vi "RIOchannelStorage.vi"(8 "Error in":errorcluster, 10 "Channel Settings":T1[][](array[typedef]), 11 "Tree DVR in":refnum<data-value>) -> (0 "Error out":errorcluster)   [LabVIEW 2014]
uses:
  Controls/RIOSettingsChannelSettings.ctl
  <vilib>/MDSplus/Classes/Tree_Class/Tree.lvclass
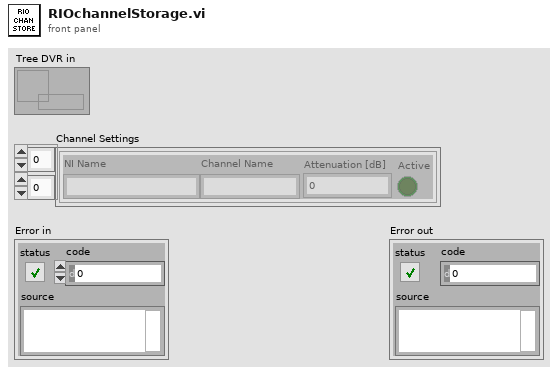
[diagram p1: front panel]
types:
  T1 = typedef "RIOSettingsChannelSettings.ctl" = cluster{"Channel Name":string, "Active":bool, "NI Name":string, "Attenuation [dB]":i32}
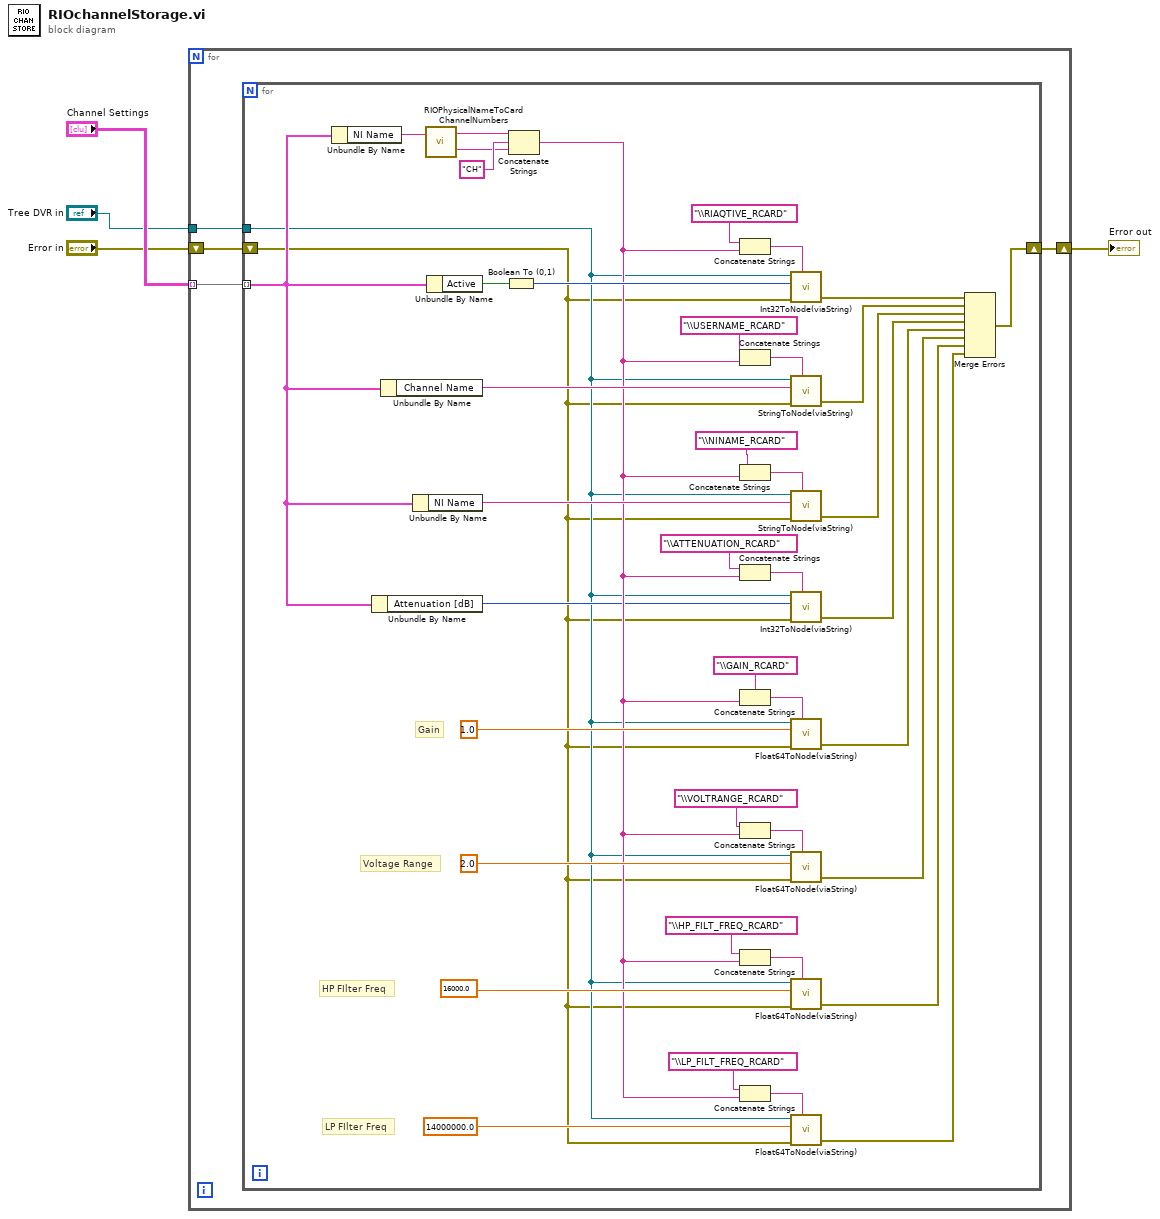
[diagram p0: block diagram]
diagram:
  n1 = for {
    tunnel: "Channel Settings" -> [w8] mode=indexing
    shift-right: [w7] -> w2
    shift-left: "Error in" -> [w5]
    tunnel: "Tree DVR in" -> [w6]
    n2 = for {
      tunnel: w8 -> [w17] mode=indexing
      tunnel: w6 -> [w15]
      shift-right: [w50] -> w7
      shift-left: w5 -> [w14]
      # "LP FIlter Freq"
      # "Voltage Range"
      # "HP FIlter Freq"
      # "Gain"
      n3 = Unbundle By Name(w17) -> ("NI Name"=w21:string)
      n4 = Unbundle By Name(w17) -> ("Attenuation [dB]"=w16:i32)
      n5 = Unbundle By Name(w17) -> ("Channel Name"=w28:string)
      n6 = Unbundle By Name(w17) -> ("NI Name"=w27:string)
      n7 = call "RIOPhysicalNameToCardChannelNumbers.vi"("Channel Name"=w21) -> ("Channel #"=w22:string, "Card #"=w23:string)  [unwired: 1 in]
      n8 = Unbundle By Name(w17) -> ("Active"=w47:bool)
      n9 = Boolean To (0,1)(Boolean=w47) -> (0, 1=w46:i16)
      n10 = Concatenate Strings(w23, "CH" ("string"), w22) -> (w18:string)
      n11 = Concatenate Strings("\\RIAQTIVE_RCARD" ("string"), w18) -> (w44:string)
      n12 = Concatenate Strings("\\USERNAME_RCARD" ("string"), w18) -> (w31:string)
      n13 = Concatenate Strings("\\NINAME_RCARD" ("string"), w18) -> (w29:string)
      n14 = Concatenate Strings("\\ATTENUATION_RCARD" ("NodePath"), w18) -> (w19:string)
      n15 = Concatenate Strings("\\GAIN_RCARD" ("string"), w18) -> (w35:string)
      n16 = Concatenate Strings("\\VOLTRANGE_RCARD" ("string"), w18) -> (w38:string)
      n17 = Concatenate Strings("\\HP_FILT_FREQ_RCARD" ("string"), w18) -> (w41:string)
      n18 = Concatenate Strings("\\LP_FILT_FREQ_RCARD" ("string"), w18) -> (w49:string)
      n19 = call "Int32ToNode(viaString).vi"("Tree DVR in"=w15, "I32 in"=w46, "error in (no error)"=w14, "NodePath"=w44) -> ("error out"=w43:errorcluster)  [unwired: 3 in]
      n20 = call "StringToNode(viaString).vi"("Tree DVR in"=w15, "String value in"=w28, "error in (no error)"=w14, "NodePath"=w31) -> ("error out"=w25:errorcluster)  [unwired: 3 in]
      n21 = call "StringToNode(viaString).vi"("Tree DVR in"=w15, "String value in"=w27, "error in (no error)"=w14, "NodePath"=w29) -> ("error out"=w26:errorcluster)  [unwired: 3 in]
      n22 = call "Int32ToNode(viaString).vi"("Tree DVR in"=w15, "I32 in"=w16, "error in (no error)"=w14, "NodePath"=w19) -> ("error out"=w9:errorcluster)  [unwired: 3 in]
      n23 = call "Float64ToNode(viaString).vi"("Tree DVR in"=w15, "DBL in"=1.0, "error in"=w14, "NodePath"=w35) -> ("error out"=w10:errorcluster)  [unwired: 3 in]
      n24 = call "Float64ToNode(viaString).vi"("Tree DVR in"=w15, "DBL in"=2.0, "error in"=w14, "NodePath"=w38) -> ("error out"=w11:errorcluster)  [unwired: 3 in]
      n25 = call "Float64ToNode(viaString).vi"("Tree DVR in"=w15, "DBL in"=16000.0, "error in"=w14, "NodePath"=w41) -> ("error out"=w12:errorcluster)  [unwired: 3 in]
      n26 = call "Float64ToNode(viaString).vi"("Tree DVR in"=w15, "DBL in"=14000000.0, "error in"=w14, "NodePath"=w49) -> ("error out"=w13:errorcluster)  [unwired: 3 in]
      n27 = Merge Errors(w43, w25, w26, w9, w10, w11, w12, w13) -> (w50:errorcluster)
    }
  }
  "Error out" <- w2
